vi "Periodic Tasks.vi"(8 "error in":errorcluster) -> ()   [LabVIEW 2014]
doc: "This VI runs in parallel to other tasks. It can contain as many user-defined periodic loops as you need. These can carry out PID or other sorts of timed response."
uses:
  <vilib>/Rock Robotics/WPI/Solenoid/WPI_SolenoidValue.ctl
  Robot Global Data.vi
  <vilib>/Rock Robotics/WPI/Solenoid/WPI_SolenoidSetEnum.vi
  <vilib>/Rock Robotics/WPI/Joystick/WPI_JoystickGetSetRefNum.vi
  <vilib>/Rock Robotics/WPI/RobotDrive/WPI_RobotDriveGetSetRefNum.vi
  <vilib>/Rock Robotics/WPI/RobotDrive/WPI_RobotDriveMecanumDrive_Cartesian.vi
  <vilib>/Rock Robotics/Network Tables/SD Write Numeric Array.vi
panel:
  in  "IntakeSpeed":dbl=0.5
  in  "error in 2":errorcluster
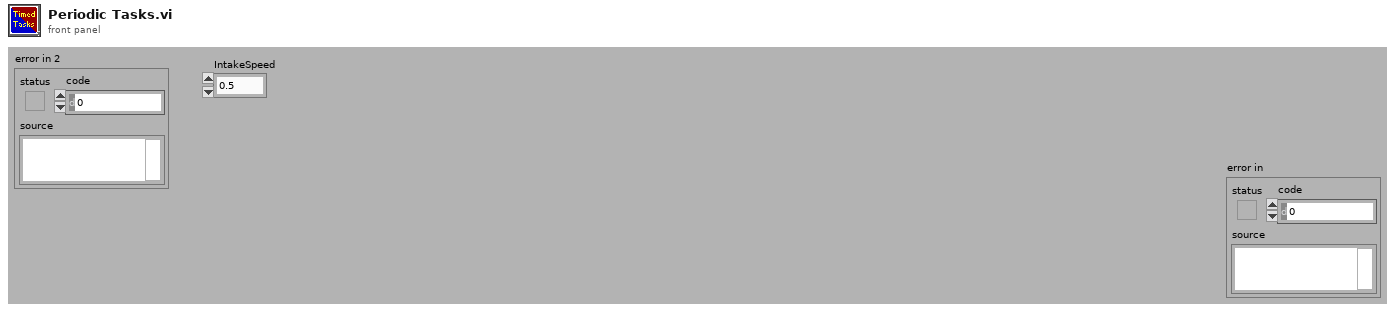
[diagram p1: front panel]
types:
  T1 = typedef "WPI_JoystickDevRef.ctl" = cluster{"Device":T2}
  T2 = typedef "WPI_JoystickDeviceEnum.ctl" = enum16{"USB 0", "USB 1", "USB 2", "USB 3", "USB 4", "USB 5"}
  T3 = typedef "WPI_RobotDriveDevRef.ctl" = cluster{"DevStatus":errorcluster, "Motors[]":T4[], "Square Inputs":bool, "Max Output":dbl}
  T4 = typedef "WPI_MotorControlDeviceRef.ctl" = cluster{"DeviceStatus":errorcluster, "Type":T5, "PWM":cluster{"Controller":T6, "PWM Channel":T7, "DeadBand":T8}, "CAN":cluster{"Device Number":u8, "Control Mode":T9, "Semaphore":T10, "Max Vout":dbl, "TalonSRX Control Mode":T11}, "Invert":bool, "TransformRef":T12, "InvTransformRef":T12}
  T5 = typedef "WPI_MotorControlType.ctl" = enum16{"PWM", "CAN", "CANTalonSRX"}
  T6 = typedef "FPGA_TypedefDigitalModule.ctl" = enum16{"Controller 1"}
  T7 = typedef "FPGA_DIOPWMChannel.ctl" = enum8{"PWM 0", "PWM 1", "PWM 2", "PWM 3", "PWM 4", "PWM 5", "PWM 6", "PWM 7", "PWM 8", "PWM 9", "PWM MXP 0", "PWM MXP 1", "PWM MXP 2", "PWM MXP 3", "PWM MXP 4", "PWM MXP 5", "PWM MXP 6", "PWM MXP 7", "PWM MXP 8", "PWM MXP 9", "Invalid"}
  T8 = typedef "WPI_PWMDeadband.ctl" = cluster{"Name":string, "maxPositivePwm":i32, "minPositivePwm":i32, "centerPwm":i32, "maxNegativePwm":i32, "minNegativePwm":i32, "angularRange":u16}
  T9 = typedef "WPI_CANJaguar_ControlMode.ctl" = enum8{"Percent VBus", "Current", "Speed", "Position", "Voltage"}
  T10 = typedef "Semaphore RefNum" = refnum<k1>
  T11 = typedef "WPI_CANTalonSRX_APIControlMode.ctl" = enum8{"Percent VBus", "Speed", "Position", "Slave", "Unchanged / Invalid"}
  T12 = typedef "WPI_PWMTransform_ConPane.ctl" = refnum<vi>
  T13 = cluster{"JoystickDevRef":T1, "RobotDriveDevRef":T3}
  T14 = typedef "WPI_SolenoidDevRef.ctl" = cluster{"DevStatus":errorcluster, "Pneumatics Control Module":u8, "Forward Solenoid Channel":T15, "Reverse Solenoid Channel":T15}
  T15 = typedef "WPI_SolenoidChannel.ctl" = enum8{"Solenoid 0", "Solenoid 1", "Solenoid 2", "Solenoid 3", "Solenoid 4", "Solenoid 5", "Solenoid 6", "Solenoid 7", "Invalid"}
  T16 = typedef "WPI_SolenoidValue.ctl" = enum16{"Off", "On", "Forward", "Reverse"}
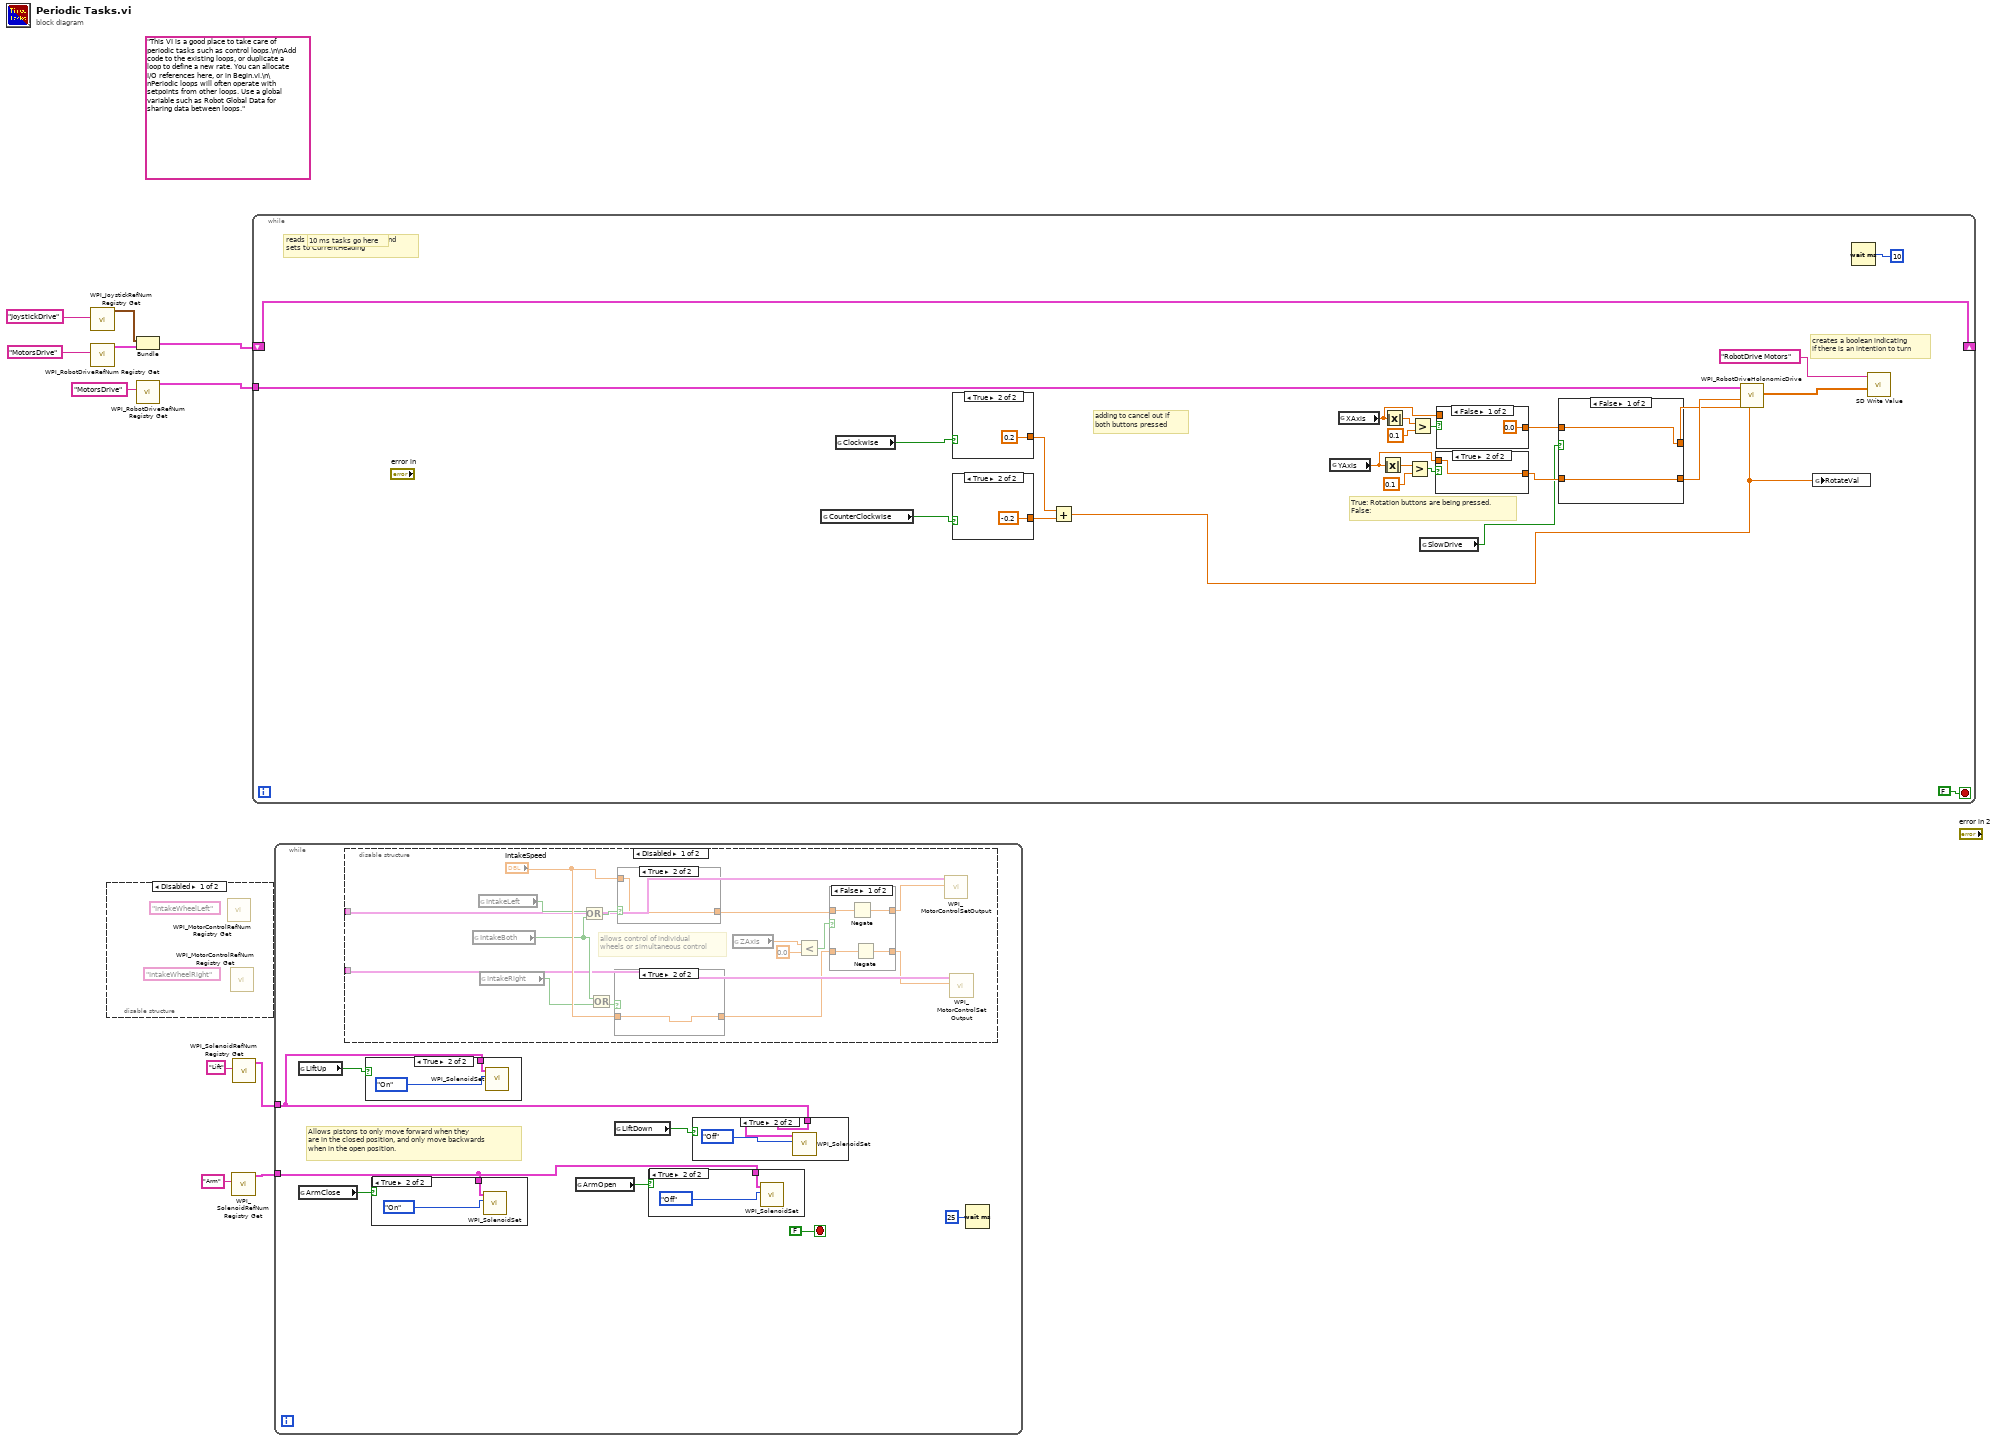
[diagram p0: block diagram]
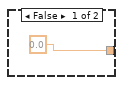
[diagram p4: hidden frame]
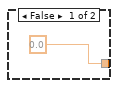
[diagram p5: hidden frame]
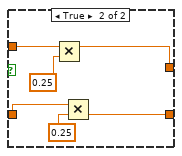
[diagram p11: hidden frame]
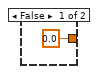
[diagram p12: hidden frame]
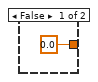
[diagram p14: hidden frame]
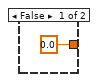
[diagram p15: hidden frame]
diagram:
  (unwired) "This VI is a good place to take care of periodic tasks such as control loops.\n\nAdd code to the existing loops, or duplicate a loop to define a new rate. You can allocate I/O references here, or in Begin.vi.\n\nPeriodic loops will often operate with setpoints from other loops. Use a global variable such as Robot Global Data for sharing data between loops."
  n1 = call <vilib>:"WPI_JoystickRefNum Registry Get.vi"("refnum name"="JoystickDrive") -> ("JoystickDevRef"=w5:T1)  [unwired: 1 in, 9 out]
  n2 = call <vilib>:"WPI_RobotDriveRefNum Registry Get.vi"("refnum name"="MotorsDrive") -> ("RobotDriveDevRef"=w4:T3)  [unwired: 1 in, 9 out]
  n3 = disable-structure shown="Disabled" {
    frame Disabled {
      (unwired) "IntakeWheelRight" ("refnum name")
      (unwired) "IntakeWheelLeft" ("refnum name")
      n4 = call <vilib>:"WPI_MotorControlRefNum Registry Get.vi"() -> ()  [unwired: 10 in, 2 out]
      n5 = call <vilib>:"WPI_MotorControlRefNum Registry Get.vi"() -> ()  [unwired: 10 in, 2 out]
    }
    frame Enabled {
    }
  }
  n6 = Bundle("JoystickDevRef"=w5, "RobotDriveDevRef"=w4) -> (w1:T13)  [unwired: 1 out]
  n7 = call <vilib>:"WPI_RobotDriveRefNum Registry Get.vi"("refnum name"="MotorsDrive") -> ("RobotDriveDevRef"=w2:T3)  [unwired: 1 in, 9 out]
  n8 = call <vilib>:"WPI_SolenoidRefNum Registry Get.vi"("refnum name"="Arm") -> ("SolenoidDevRef"=w9:T14)  [unwired: 9 in, 1 out]
  n9 = call <vilib>:"WPI_SolenoidRefNum Registry Get.vi"("refnum name"="Lift") -> ("SolenoidDevRef"=w8:T14)  [unwired: 9 in, 1 out]
  n10 = while {
    shift-right: [w29] -> _
    shift-left: w1 -> [w29]
    tunnel: w2 -> [w26]
    stop <- FALSE stop-if-true
    # "True: Rotation buttons are being pressed.\nFalse:"
    # "creates a boolean indicating \nif there is an intention to turn"
    # "adding to cancel out if \nboth buttons pressed"
    # "reads the current gyro angle and \nsets to CurrentHeading"
    # "10 ms tasks go here"
    n11 = global read "Robot Global Data.vi" "CounterClockwise"() -> (w32:bool)
    n12 = global read "Robot Global Data.vi" "Clockwise"() -> (w33:bool)
    n13 = case shown="True" w33 {
      tunnel: [0.0 0.2] -> w31
      frame False {
      }
      frame True {
      }
    }
    n14 = case shown="True" w32 {
      tunnel: [0.0 -0.2] -> w30
      frame False {
      }
      frame True {
      }
    }
    n15 = Add(x=w31, y=w30) -> (x+y=w12:dbl)
    n16 = global read "Robot Global Data.vi" "YAxis"() -> (w18:dbl)
    n17 = global read "Robot Global Data.vi" "XAxis"() -> (w19:dbl)
    n18 = Absolute Value(x=w18) -> (abs(x)=w21:dbl)
    n19 = Absolute Value(x=w19) -> (abs(x)=w22:dbl)
    n20 = Greater?(x=w21, y=0.1) -> (0:w25:bool)
    n21 = Greater?(x=w22, y=0.1) -> (0:w24:bool)
    n22 = global read "Robot Global Data.vi" "SlowDrive"() -> (w13:bool)
    n23 = case shown="True" w25 {
      tunnel: w18 -> [_ w45]
      tunnel: [0.0 ("YAxis") w45] -> w17
      frame False {
      }
      frame True {
      }
    }
    n24 = case shown="False" w24 {
      tunnel: w19 -> [_ w47]
      tunnel: [0.0 ("XAxis") w47] -> w14
      frame False {
      }
      frame True {
      }
    }
    n25 = case shown="False" w13 {
      tunnel: w17 -> [w36 w39]
      tunnel: [w36 w40] -> w16
      tunnel: [w37 w42] -> w15
      tunnel: w14 -> [w37 w43]
      frame False {
      }
      frame True {
        n26 = Multiply(x=w43, y=0.25) -> (x*y=w42:dbl)
        n27 = Multiply(x=w39, y=0.25) -> (x*y=w40:dbl)
      }
    }
    n28 = call-poly <vilib>:"WPI_RobotDriveHolonomicDrive.vi"("Rotation"=w12, "Y"=w16, "X"=w15, "RobotDriveDevRef"=w26) -> ("Motor Values"=w27:dbl[])  [unwired: 5 in, 2 out]
    n29 = global write "Robot Global Data.vi" "RotateVal"(w12) -> ()
    n30 = Wait (ms)(milliseconds to wait=u32 10) -> ()  [unwired: 1 out]
    n31 = call-poly <vilib>:"SD Write Value.vi"("Numeric Array"=w27, "Name"="RobotDrive Motors") -> ()  [unwired: 8 in, 2 out]
  }
  n32 = while {
    tunnel: w9 -> [w53]
    tunnel: w8 -> [w52]
    stop <- FALSE stop-if-true
    # "Allows pistons to only move forward when they \nare in the closed position, and only move backwards \nwhen in the open position."
    n33 = global read "Robot Global Data.vi" "LiftUp"() -> (w56:bool)
    n34 = global read "Robot Global Data.vi" "ArmClose"() -> (w59:bool)
    n35 = disable-structure shown="Disabled" {
      disable-tunnel: _ -> [w68 _]
      disable-tunnel: _ -> [w67 _]
      frame Disabled {
        # "allows control of individual \nwheels or simultaneous control"
        n36 = global read "Robot Global Data.vi" "IntakeBoth"() -> (w70:bool)
        n37 = global read "Robot Global Data.vi" "IntakeLeft"() -> (w69:bool)
        n38 = global read "Robot Global Data.vi" "IntakeRight"() -> (w71:bool)
        n39 = Or(x=w69, y=w70) -> (x .or. y?=w73:bool)
        n40 = Or(x=w70, y=w71) -> (x .or. y?=w72:bool)
        n41 = case shown="True" w72 {
          tunnel: [0.0 ("IntakeSpeed") w82] -> w61
          tunnel: "IntakeSpeed" -> [_ w82]
          frame False {
          }
          frame True {
          }
        }
        n42 = case shown="True" w73 {
          tunnel: [0.0 ("IntakeSpeed") w84] -> w63
          tunnel: "IntakeSpeed" -> [_ w84]
          frame False {
          }
          frame True {
          }
        }
        n43 = global read "Robot Global Data.vi" "ZAxis"() -> (w65:dbl)
        n44 = Less?(x=w65, y=0.0) -> (x < y?=w66:bool)
        n45 = case shown="False" w66 {
          tunnel: w63 -> [w78 w80]
          tunnel: [w76 w80] -> w62
          tunnel: w61 -> [w77 w79]
          tunnel: [w75 w79] -> w60
          frame False {
            n46 = Negate(x=w78) -> (-x=w76:dbl)
            n47 = Negate(x=w77) -> (-x=w75:dbl)
          }
          frame True {
          }
        }
        n48 = call <vilib>:"WPI_MotorControlSetOutput.vi"("Output"=w62, "MotorControlDevRef"=w67) -> ()  [unwired: 7 in, 3 out]
        n49 = call <vilib>:"WPI_MotorControlSetOutput.vi"("Output"=w60, "MotorControlDevRef"=w68) -> ()  [unwired: 7 in, 3 out]
      }
      frame Enabled {
      }
    }
    n50 = case shown="True" w56 {
      tunnel: w52 -> [_ w92]
      frame False {
      }
      frame True {
        n51 = call-poly <vilib>:"WPI_SolenoidSet.vi"("Value"=WPI_SolenoidValue."On", "SolenoidDevRef"=w92) -> ()  [unwired: 8 in, 2 out]
      }
    }
    n52 = case shown="True" w59 {
      tunnel: w53 -> [_ w89]
      frame False {
      }
      frame True {
        n53 = call-poly <vilib>:"WPI_SolenoidSet.vi"("Value"=WPI_SolenoidValue."On", "SolenoidDevRef"=w89) -> ()  [unwired: 8 in, 2 out]
      }
    }
    n54 = global read "Robot Global Data.vi" "ArmOpen"() -> (w54:bool)
    n55 = global read "Robot Global Data.vi" "LiftDown"() -> (w55:bool)
    n56 = case shown="True" w54 {
      tunnel: w53 -> [_ w85]
      frame False {
      }
      frame True {
        n57 = call-poly <vilib>:"WPI_SolenoidSet.vi"("Value"=WPI_SolenoidValue."Off", "SolenoidDevRef"=w85) -> ()  [unwired: 8 in, 2 out]
      }
    }
    n58 = case shown="True" w55 {
      tunnel: w52 -> [_ w88]
      frame False {
      }
      frame True {
        n59 = call-poly <vilib>:"WPI_SolenoidSet.vi"("Value"=WPI_SolenoidValue."Off", "SolenoidDevRef"=w88) -> ()  [unwired: 8 in, 2 out]
      }
    }
    n60 = Wait (ms)(milliseconds to wait=u32 25) -> ()  [unwired: 1 out]
  }
